vi "MCL Wfma Stop.vi"(11 "handle":i32) -> (3 "function return":i32)   [LabVIEW 2017, in "Madlib.lvlib"]
doc: "MADLIB_API int MCL_WfmaStop(int handle);"
uses:
  Madlib.lvlib
  Madlib.dll
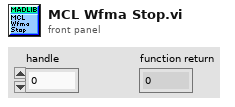
[diagram p1: front panel]
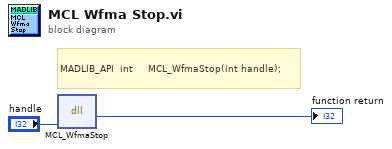
[diagram p0: block diagram]
diagram:
  # "MADLIB_API  int     MCL_WfmaStop(int handle);"
  n1 = dll-call lib="C:/Users/francesco/dev/pump-probe/Piezo/lvlib/Madlib.*" fn="MCL_WfmaStop"("handle"="handle") -> (→"function return":i32)  [unwired: 4 in, 2 out]
